vi "MSDateienSchicken02-15.vi"(1 "MSNummer":i32, 2 "MSa?":bool=TRUE, 3 "Dateipfad:fromcriordy":path, 4 "Dateipfad:fromcriocmd":path) -> ()   [LabVIEW 2010]
uses:
  GVZeitenZyklen.vi
  GVProbenvol.vi
  GVVentilposition.vi
  <vilib>/addons/internet/NI_InternetTK_FTP_VIs.lvlib
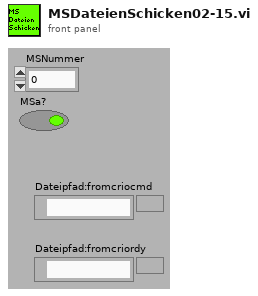
[diagram p1: front panel]
types:
  T1 = enum16{"open", "replace", "create", "open or create", "replace or create", "replace or create with confirmation"}
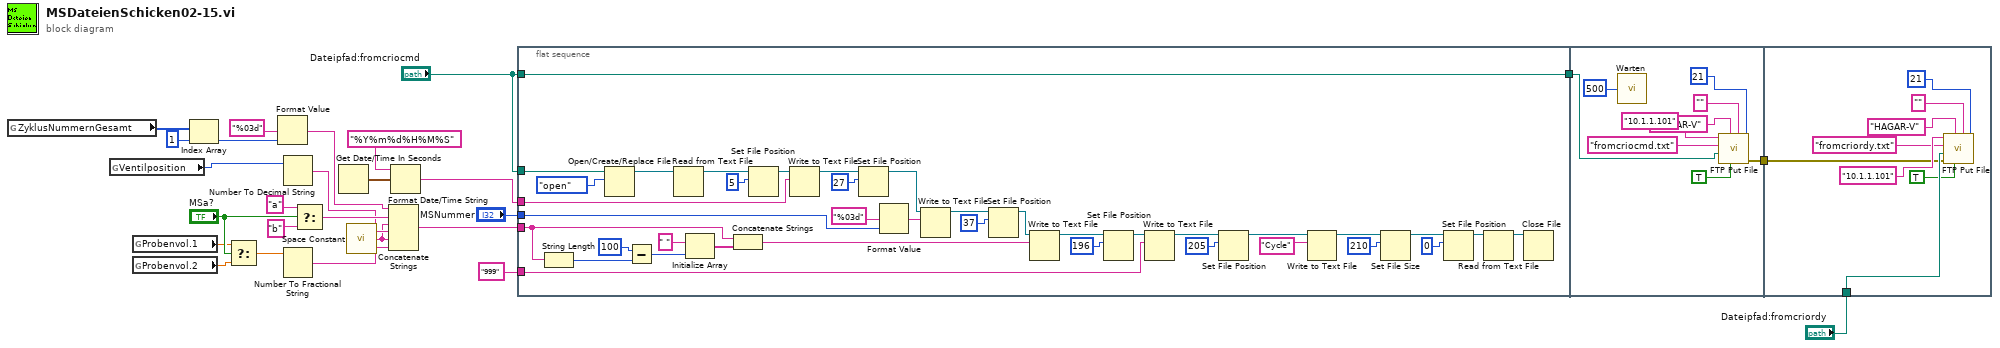
[diagram p0: block diagram]
diagram:
  n1 = global read "GVZeitenZyklen.vi" "ZyklusNummernGesamt"() -> (w19:i32[])
  n2 = global read "GVVentilposition.vi" "Ventilposition"() -> (w1:i32)
  n3 = global read "GVProbenvol.vi" "Probenvol.1"() -> (w3:dbl)
  n4 = global read "GVProbenvol.vi" "Probenvol.2"() -> (w2:dbl)
  n5 = Index Array(array=w19, index=1 ("Index")) -> (element=w15:i32)
  n6 = Select(t=w3, s="MSa?", f=w2) -> (s? t:f=w5:dbl)
  n7 = Format Value(format string="%03d" ("Format-String"), value (0)=w15) -> (output string=w11:string)  [unwired: 1 in]
  n8 = Number To Decimal String(number=w1) -> (decimal integer string=w9:string)  [unwired: 1 in]
  n9 = Number To Fractional String(number=w5) -> (F-format string=w4:string)  [unwired: 3 in]
  n10 = Select(t="a", s="MSa?", f="b") -> (s? t:f=w10:string)
  n11 = Get Date/Time In Seconds() -> (seconds since 1Jan1904=w22:timestamp)
  n12 = call <vilib>:"Space Constant.vi"() -> ("String"=w8:string)
  n13 = Concatenate Strings(w11, w10, w8, w9, w8, w4) -> (w7:string)
  n14 = Format Date/Time String(time format string (%c)="%Y%m%d%H%M%S" ("Zeitformatierungs-String (%c)"), seconds (now)=w22) -> (date/time string=w21:string)  [unwired: 1 in]
  n15 = flat-sequence {
    tunnel: [w64] -> w17
    tunnel: "999" ("Speicherlänge") -> [w30]
    tunnel: w7 -> [w29]
    tunnel: w21 -> [w28]
    tunnel: "MSNummer" -> [w27]
    tunnel: "Dateipfad:fromcriocmd" -> [w64]
    tunnel: "Dateipfad:fromcriocmd" -> [w31]
    tunnel: [w65] -> w16
    tunnel: w17 -> [w70]
    tunnel: "Dateipfad:fromcriordy" -> [w78]
    tunnel: w16 -> [w74]
    frame #0 {
      n16 = String Length(string=w29) -> (length=w58:i32)
      n17 = Open/Create/Replace File(file path (use dialog)=w31, operation (0:open)=T1."open" ("Operation (0:Öffnen)")) -> (refnum out=w34:refnum<file>)  [unwired: 4 in, 2 out]
      n18 = Subtract(x=100, y=w58) -> (x-y=w60:i32)
      n19 = Read from Text File(file (use dialog)=w34) -> (refnum out=w35:refnum<file>)  [unwired: 3 in, 3 out]
      n20 = Initialize Array(" ", w60) -> (w62:string[])
      n21 = Concatenate Strings(w29, w62) -> (w63:string)
      n22 = Set File Position(offset (in bytes) (0)=i64 5 ("Offset (in Byte) (0)"), refnum=w35) -> (refnum out=w41:refnum<file>)  [unwired: 2 in, 1 out]
      n23 = Write to Text File(file (use dialog)=w41, text=w28) -> (refnum out=w43:refnum<file>)  [unwired: 2 in, 2 out]
      n24 = Set File Position(offset (in bytes) (0)=i64 27 ("Offset (in Byte) (0)"), refnum=w43) -> (refnum out=w42:refnum<file>)  [unwired: 2 in, 1 out]
      n25 = Format Value(format string="%03d" ("Format-String"), value (0)=w27) -> (output string=w57:string)  [unwired: 1 in]
      n26 = Write to Text File(file (use dialog)=w42, text=w57) -> (refnum out=w44:refnum<file>)  [unwired: 2 in, 2 out]
      n27 = Set File Position(offset (in bytes) (0)=i64 37 ("Offset (in Byte) (0)"), refnum=w44) -> (refnum out=w45:refnum<file>)  [unwired: 2 in, 1 out]
      n28 = Write to Text File(file (use dialog)=w45, text=w63) -> (refnum out=w46:refnum<file>)  [unwired: 2 in, 2 out]
      n29 = Set File Position(offset (in bytes) (0)=i64 196 ("Offset (in Byte) (0)"), refnum=w46) -> (refnum out=w47:refnum<file>)  [unwired: 2 in, 1 out]
      n30 = Write to Text File(file (use dialog)=w47, text=w30) -> (refnum out=w53:refnum<file>)  [unwired: 2 in, 2 out]
      n31 = Set File Position(offset (in bytes) (0)=i64 205 ("Offset (in Byte) (0)"), refnum=w53) -> (refnum out=w52:refnum<file>)  [unwired: 2 in, 1 out]
      n32 = Write to Text File(file (use dialog)=w52, text="Cycle") -> (refnum out=w54:refnum<file>)  [unwired: 2 in, 2 out]
      n33 = Set File Size(6:i64 210 ("Größe (in Byte)"), 7:w54) -> (3:w49:refnum<file>)  [unwired: 1 in, 1 out]
      n34 = Set File Position(offset (in bytes) (0)=i64 0 ("Offset (in Byte) (0)"), refnum=w49) -> (refnum out=w40:refnum<file>)  [unwired: 2 in, 1 out]
      n35 = Read from Text File(file (use dialog)=w40) -> (refnum out=w50:refnum<file>)  [unwired: 3 in, 3 out]
      n36 = Close File(refnum=w50) -> ()  [unwired: 1 in, 2 out]
    }
    frame #1 {
      n37 = call "Warten"("Count(mSec)"=u32 500 ("Zu wartende ms")) -> ()  [unwired: 1 out]
      n38 = call <vilib>:"FTP Put File.vi"("remote port (21)"=u16 21, "password"="" ("user"), "binary (F)"=TRUE, "user"="HAGAR-V", "local path"=w70, "remote path"="fromcriocmd.txt", "host"="10.1.1.101") -> ("error out"=w65:errorcluster)  [unwired: 3 in, 1 out]
    }
    frame #2 {
      n39 = call <vilib>:"FTP Put File.vi"("remote port (21)"=u16 21, "password"="" ("user"), "binary (F)"=TRUE, "user"="HAGAR-V", "error in (no error)"=w74, "local path"=w78, "remote path"="fromcriordy.txt", "host"="10.1.1.101") -> ()  [unwired: 2 in, 2 out]
    }
  }
